vi "ClusterLoad.vi"(11 "Experiment State":T1={"Send Trigger 3"=FALSE, "error"={"status"=TRUE, "code"=-200088, "source"="DAQmx Wait Until Done.vi:3580005<append>\n"}, "Tasks"={"Fiber15 MP Task"="MyVoltageTask", "Read Slow AI"="", "Fiber Bank DIO"="", "Fiber7 MP Task"="MyVoltageTask", "TaskArray"=["", "", ""]}, "Channels"={"6133 Channels"=[["DAQ1/ai0", "DAQ1/ai1", "DAQ1/ai2", "DAQ1/ai3", "DAQ1/ai4", "DAQ1/ai5", "DAQ1/ai6", "DAQ1/ai7"], ["DAQ2/ai0", "DAQ2/ai1", "DAQ2/ai2", "DAQ2/ai3", "DAQ2/ai4", "DAQ2/ai5", "DAQ2/ai6", "DAQ2/ai7"], ["DAQ3/ai0", "DAQ3/ai1", "DAQ3/ai2", "DAQ3/ai3", "DAQ3/ai4", "DAQ3/ai5", "DAQ3/ai6", "DAQ3/ai7"]], "Edge Type"=10280, "Samples Per Channel"=[50, 50, 25], "#Pre-Trigger Samples"=[25, 25, 0], "Sample Rate 2.5Ms/s Max"=[2500000.0, 2500000.0, 2500000.0], "Trigger Sources"=["PXI_Star2", "PXI_Star3", "PXI_Star4"], "Voltage Ranges"=[[10.0, 10.0, 10.0, 10.0, 10.0, 10.0, 10.0, 10.0], [10.0, 10.0, 10.0, 10.0, 10.0, 10.0, 10.0, 10.0], [10.0, 10.0, 10.0, 10.0, 10.0, 10.0, 10.0, 10.0]], "Channel Names"=[["1", "2", "3", "4", "5", "6", "7", "8"], ["9", "10", "11", "12", "13", "14", "15", "16"], ["17", "18", "19", "20", "21", "22", "23", "24"]], "Active"=[[TRUE, TRUE, TRUE, TRUE, TRUE, TRUE, TRUE, TRUE], [TRUE, TRUE, TRUE, TRUE, TRUE, TRUE, TRUE, TRUE], [TRUE, TRUE, TRUE, TRUE, TRUE, TRUE, TRUE, TRUE]], "Pre-Trigger Time"=[9.999999999999999e-06, 9.999999999999999e-06, 0.0], "Total Sample Time"=[1.9999999999999998e-05, 1.9999999999999998e-05, 9.999999999999999e-06], "Sampling Times"=[]}, "Dev 10 DIO"="", "Dev5"="", "Fiber Triggers 2"=[{"Delay (s)"=9.999999999999999e-05, "Pulse width (s)"=9.999999999999999e-05, "Active"=TRUE, "Channel Name"="9", "counter"="Timing2/ctr0"}, {"Delay (s)"=9.999999999999999e-05, "Pulse width (s)"=9.999999999999999e-05, "Active"=TRUE, "Channel Name"="10", "counter"="Timing2/ctr1"}, {"Delay (s)"=9.999999999999999e-05, "Pulse width (s)"=9.999999999999999e-05, "Active"=TRUE, "Channel Name"="11", "counter"="Timing2/ctr2"}, {"Delay (s)"=9.999999999999999e-05, "Pulse width (s)"=9.999999999999999e-05, "Active"=TRUE, "Channel Name"="12", "counter"="Timing2/ctr3"}, {"Delay (s)"=9.999999999999999e-05, "Pulse width (s)"=9.999999999999999e-05, "Active"=TRUE, "Channel Name"="13", "counter"="Timing2/ctr4"}, {"Delay (s)"=9.999999999999999e-05, "Pulse width (s)"=9.999999999999999e-05, "Active"=TRUE, "Channel Name"="14", "counter"="Timing2/ctr5"}, {"Delay (s)"=0.00019999999999999998, "Pulse width (s)"=9.999999999999999e-05, "Active"=TRUE, "Channel Name"="15", "counter"="Timing2/ctr6"}, {"Delay (s)"=9.999999999999999e-05, "Pulse width (s)"=9.999999999999999e-05, "Active"=TRUE, "Channel Name"="16", "counter"="Timing2/ctr7"}], "MP7"=FALSE, "MP15"=FALSE, "PXI Slot 2"={"PXI Slot 2 Handle"="Sync", "source terminal"="GlobalSoftwareTrigger"}, "# of Control DIOs"=0, "Bank DIO Settings"=[], "Purge Duration (s)"=5, "Interlock Override"=FALSE, "Current Raw Voltages, Slot &"=[], "Bank Control"={"Bank Enables"={"Gun1 Enable"=FALSE, "Gun2 Enable"=FALSE, "InnerSol Enable"=FALSE, "OuterSol1 Enable"=FALSE, "Outer2 Enable"=FALSE, "Gun3 Enable"=FALSE}, "Voltages"={"Gun1 Voltage"=0.0, "Gun2 Voltage"=0.0, "Gun3 Voltage"=0.0, "InnerSol Voltage"=0.0, "OuterSol1 Voltage"=0.0, "OuterSol2 Voltage"=0.0}, "Set Points"={"Gun1 Setpoint"=0.0, "Gun2 Setpoint"=0.0, "Gun3 Setpoint"=0.0, "InnerSol Setpoint"=0.0, "OuterSol1 Setpoint"=0.0, "OuterSol2 Setpoint"=0.0}}, "Waveform Data"=[], "Next Shot#"="6", "Slot 7, Last Shot Scaled Voltages"=[], "Data Run Description"="", "Next Shot Data"=[], "Headers"=[], "Html Shot Log View"=FALSE, "ShotLog Headers"=path "", "ShotLog Data"=path "", "Enable Bank Control"=FALSE, "6602  Slot8"={"Slot 8 Trigger Source"="/Timing1/PXI_Star", "Slot 8 Clock Source"="/Timing1/80MHzTimebase", "Trigger Channel Tasks"=["", "", "", "", "", "", "", ""]}, "6602  Slot 9"={"Slot 9 Clock Source"="/Timing2/80MHzTimebase", "Slot 9 Trigger Source"="/Timing2/PXI_Star", "Trigger Channel Tasks"=["", "", "", "", "", "", "", ""]}, "Fiber Triggers"=[{"Delay (s)"=9.999999999999999e-05, "Pulse width (s)"=0.0, "Active"=TRUE, "Channel Name"="1", "counter"="Timing1/ctr0"}, {"Delay (s)"=9.999999999999999e-05, "Pulse width (s)"=9.999999999999999e-05, "Active"=TRUE, "Channel Name"="2", "counter"="Timing1/ctr1"}, {"Delay (s)"=9.999999999999999e-05, "Pulse width (s)"=9.999999999999999e-05, "Active"=TRUE, "Channel Name"="3", "counter"="Timing1/ctr2"}, {"Delay (s)"=0.0, "Pulse width (s)"=9.999999999999999e-05, "Active"=TRUE, "Channel Name"="4", "counter"="Timing1/ctr3"}, {"Delay (s)"=9.999999999999999e-05, "Pulse width (s)"=9.999999999999999e-05, "Active"=TRUE, "Channel Name"="5", "counter"="Timing1/ctr4"}, {"Delay (s)"=9.999999999999999e-05, "Pulse width (s)"=9.999999999999999e-05, "Active"=TRUE, "Channel Name"="6", "counter"="Timing1/ctr5"}, {"Delay (s)"=9.999999999999999e-05, "Pulse width (s)"=9.999999999999999e-05, "Active"=TRUE, "Channel Name"="7", "counter"="Timing1/ctr6"}, {"Delay (s)"=9.999999999999999e-05, "Pulse width (s)"=9.999999999999999e-05, "Active"=TRUE, "Channel Name"="8", "counter"="Timing1/ctr7"}], "System Message"="21:40:10 - Program Loaded - Idle\r\n", "Shot Notes"="Testing MDSplus \n\n"} {"Fiber Triggers"."Pulse width (s)" format="%.3p"; "Fiber Triggers"."Delay (s)" format="%.3p"; "Current Raw Voltages, Slot &" format="%0.2f"; "Fiber Triggers 2"."Pulse width (s)" format="%.3p"; "Fiber Triggers 2"."Delay (s)" format="%.3p"; "Channels"."Total Sample Time" format="%#_6f"; "Channels"."Pre-Trigger Time" format="%#_6f"; "Channels"."Sample Rate 2.5Ms/s Max" format="%#_3p"; "Channels"."Edge Type" items=["Rising"=10280, "Falling"=10171]}) -> ()   [LabVIEW 2013]
uses:
  Controls/ExperimentStateCluster.ctl
panel:
  in  "Load":bool
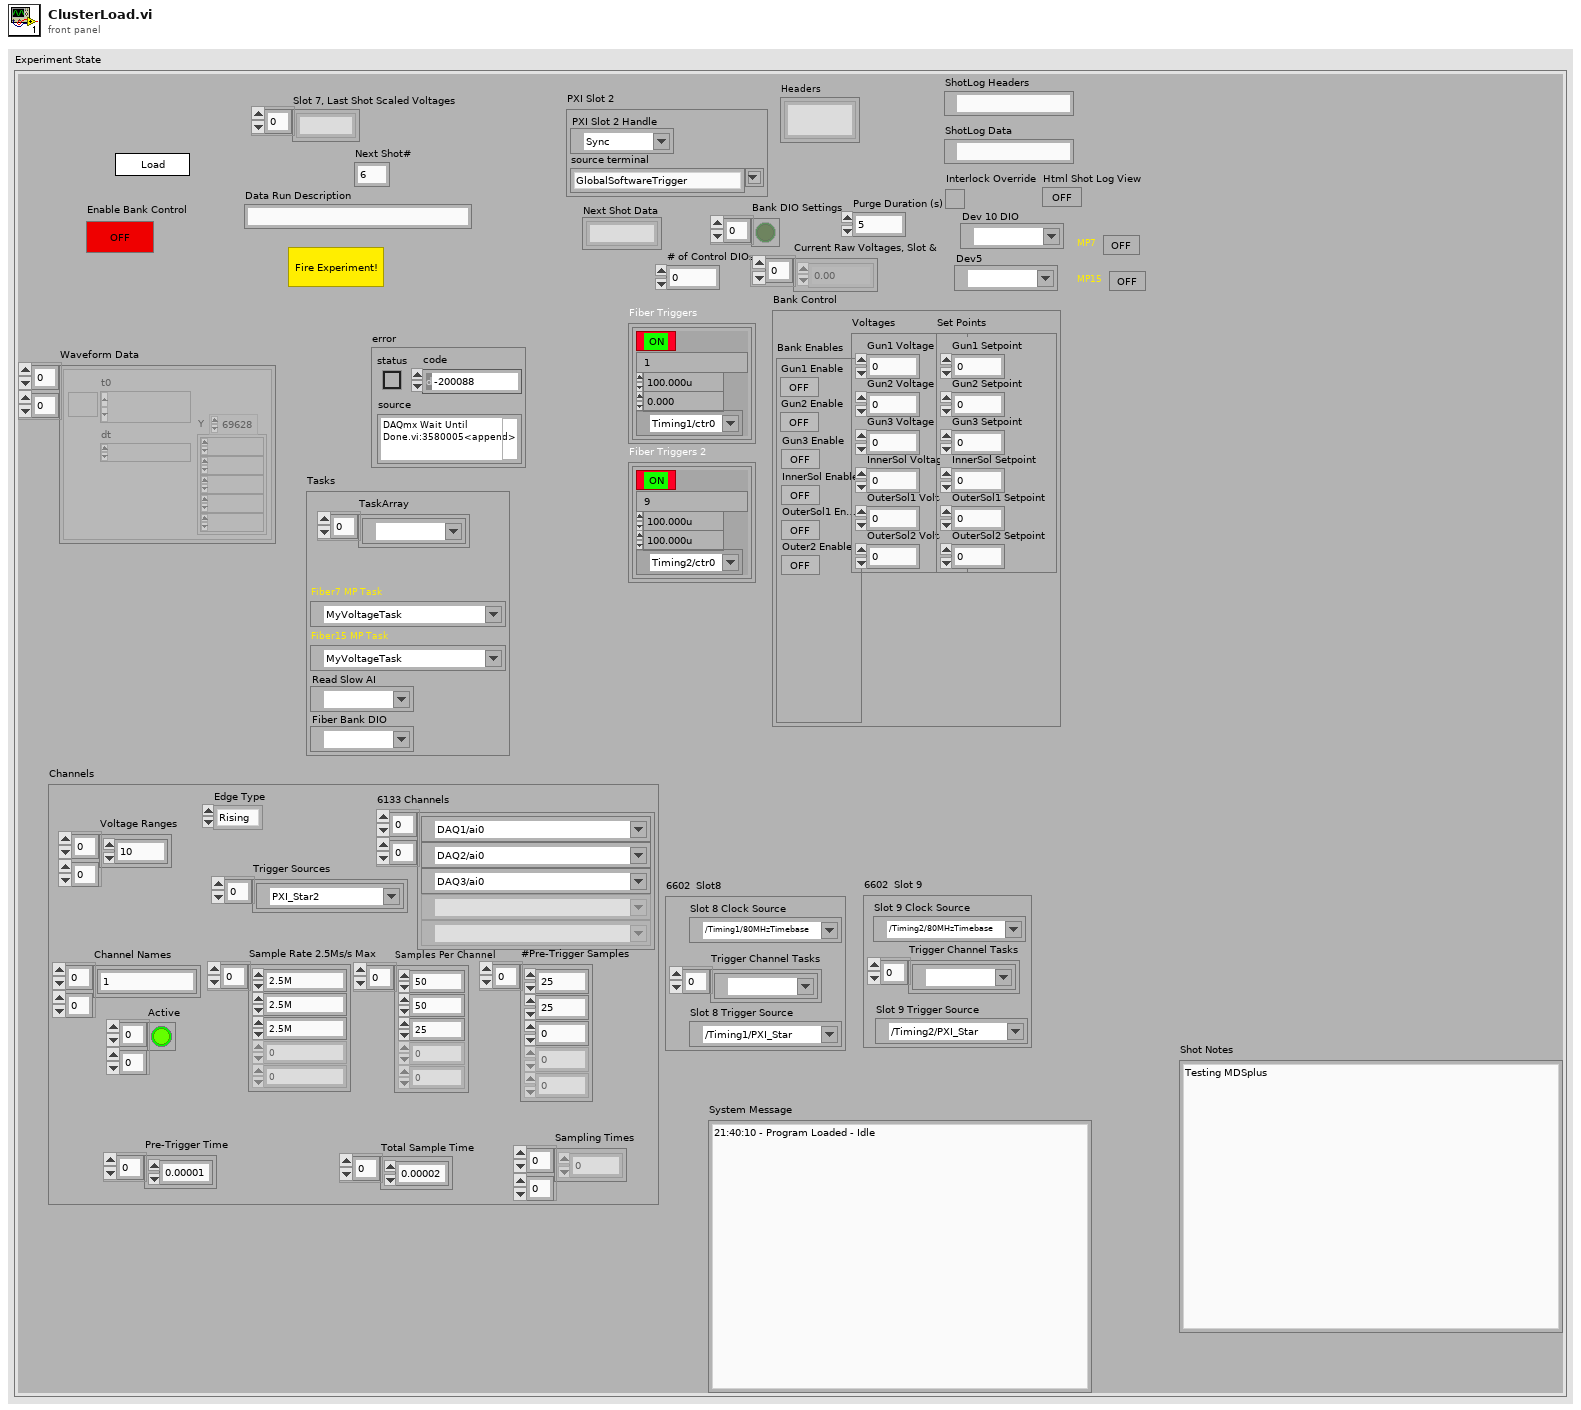
[diagram p1: front panel]
types:
  T1 = typedef "ExperimentStateCluster.ctl" = cluster{"Send Trigger 3":bool, "error":errorcluster, "Tasks":cluster{"Fiber15 MP Task":refnum<k21>, "Read Slow AI":refnum<k21>, "Fiber Bank DIO":refnum<k21>, "Fiber7 MP Task":refnum<k21>, "TaskArray":refnum<k21>[]}, "Channels":cluster{"6133 Channels":tag[][], "Edge Type":i32, "Samples Per Channel":i32[], "#Pre-Trigger Samples":u32[], "Sample Rate 2.5Ms/s Max":dbl[], "Trigger Sources":tag[], "Voltage Ranges":dbl[][], "Channel Names":string[][], "Active":bool[][], "Pre-Trigger Time":dbl[], "Total Sample Time":dbl[], "Sampling Times":dbl[][]}, "Dev 10 DIO":refnum<k21>, "Dev5":refnum<k21>, "Fiber Triggers 2":cluster{"Delay (s)":dbl, "Pulse width (s)":dbl, "Active":bool, "Channel Name":string, "counter":tag}[], "MP7":bool, "MP15":bool, "PXI Slot 2":cluster{"PXI Slot 2 Handle":refnum<k15>, "source terminal":string}, "# of Control DIOs":i32, "Bank DIO Settings":bool[], "Purge Duration (s)":u32, "Interlock Override":bool, "Current Raw Voltages, Slot &":dbl[], "Bank Control":cluster{"Bank Enables":cluster{"Gun1 Enable":bool, "Gun2 Enable":bool, "InnerSol Enable":bool, "OuterSol1 Enable":bool, "Outer2 Enable":bool, "Gun3 Enable":bool}, "Voltages":cluster{"Gun1 Voltage":dbl, "Gun2 Voltage":dbl, "Gun3 Voltage":dbl, "InnerSol Voltage":dbl, "OuterSol1 Voltage":dbl, "OuterSol2 Voltage":dbl}, "Set Points":cluster{"Gun1 Setpoint":dbl, "Gun2 Setpoint":dbl, "Gun3 Setpoint":dbl, "InnerSol Setpoint":dbl, "OuterSol1 Setpoint":dbl, "OuterSol2 Setpoint":dbl}}, "Waveform Data":waveform(dbl)[][], "Next Shot#":string, "Slot 7, Last Shot Scaled Voltages":string[], "Data Run Description":string, "Next Shot Data":string[], "Headers":string[], "Html Shot Log View":bool, "ShotLog Headers":path, "ShotLog Data":path, "Enable Bank Control":bool, "6602  Slot8":cluster{"Slot 8 Trigger Source":tag, "Slot 8 Clock Source":tag, "Trigger Channel Tasks":refnum<k21>[]}, "6602  Slot 9":cluster{"Slot 9 Clock Source":tag, "Slot 9 Trigger Source":tag, "Trigger Channel Tasks":refnum<k21>[]}, "Fiber Triggers":cluster{"Delay (s)":dbl, "Pulse width (s)":dbl, "Active":bool, "Channel Name":string, "counter":tag}[], "System Message":string, "Shot Notes":string}
  T2 = enum16{"open", "open or create", "create or replace", "create", "open (read only)"}
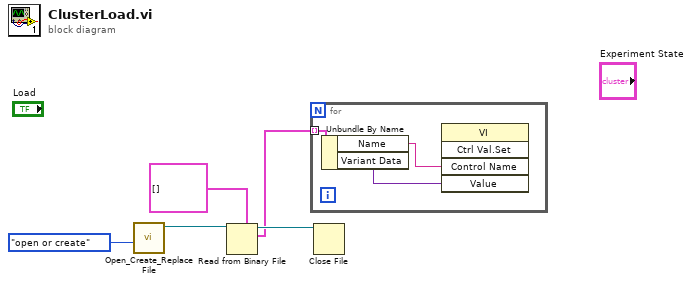
[diagram p0: block diagram]
diagram:
  n1 = call <vilib>:"Open_Create_Replace File.vi"("function (open:0)"=T2."open or create") -> ("refnum"=w5:refnum<file>)  [unwired: 7 in, 3 out]
  n2 = Read from Binary File(5:cluster{"Name":string, "Variant Data":variant}[] [] ("Control Value:Get All"), 11:w5) -> (2:w2:cluster{"Name":string, "Variant Data":variant}[], 3:w4:refnum<file>)  [unwired: 4 in, 2 out]
  n3 = for {
    tunnel: w2 -> [w8] mode=indexing
    n4 = Unbundle By Name(w8) -> ("Name"=w7:string, "Variant Data"=w6:variant)
    n5 = invoke class="VI" method="Ctrl Val.Set"("Control Name"=w7, "Value"=w6) -> ()  [unwired: 3 in, 5 out]
  }
  n6 = Close File(refnum=w4) -> ()  [unwired: 1 in, 2 out]
